vi "Close.vi"(8 "error in (no error)":errorcluster, 11 "DIO Ref In":T1) -> (0 "error out":errorcluster)   [LabVIEW 2021, in "DIO.lvlib"]
doc: "Closes the reference to one or more digital I/O channels, sets the logic levels of all output channels to low, and disables all output channels."
uses:
  <vilib>/myRIO/Instrument Drivers/Onboard IO/DIO/DIO.lvlib
  <vilib>/myRIO/Instrument Drivers/Onboard IO/DIO/typedefs/DIO Reference.ctl
  <vilib>/myRIO/Common/Instrument Driver Framework/Utilities/typedefs/myRIO Generic Hardware Reference.ctl
  <vilib>/myRIO/Common/Instrument Driver Framework/Utilities/typedefs/Hardware Version Enum.ctl
  <vilib>/myRIO/Common/Instrument Driver Framework/Utilities/typedefs/myRIO v1.0 Reference.ctl
  <vilib>/myRIO/Common/Instrument Driver Framework/Utilities/typedefs/Generic FPGA Reference.ctl
  <vilib>/myRIO/Common/Instrument Driver Framework/myRIO v1.0/DIO/typedefs/DIO Channels List.ctl
  <vilib>/myRIO/Common/Instrument Driver Framework/myRIO v1.0/DIO/typedefs/DIO Channels Enum.ctl
  <vilib>/myRIO/Common/Instrument Driver Framework/myRIO v1.0/DIO/vis/myRIO v1.0 Unreserve DIO.vi
  <vilib>/myRIO/Common/Instrument Driver Framework/roboRIO v1.0/DIO/vis/roboRIO v1.0 Unreserve DIO.vi
  <vilib>/myRIO/Common/Instrument Driver Framework/ELVIS III v1.0/DIO/vis/ELVIS III v1.0 Unreserve DIO.vi
  <vilib>/myRIO/Common/Instrument Driver Framework/myRIO v1.0/DIO/vis/myRIO v1.0 Build MUX Configuration DIO.vi
  <vilib>/myRIO/Common/Instrument Driver Framework/myRIO v1.0/Resource Manager/vis/myRIO v1.0 Unreserve Channel List.vi
  <vilib>/myRIO/Common/Instrument Driver Framework/roboRIO v1.0/Resource Manager/vis/roboRIO v1.0 Unreserve Channel List.vi
  <vilib>/myRIO/Common/Instrument Driver Framework/roboRIO v1.0/DIO/vis/roboRIO v1.0 Build MUX Configuration DIO.vi
  <vilib>/myRIO/Common/Instrument Driver Framework/ELVIS III v1.0/DIO/vis/ELVIS III v1.0 Build MUX Configuration DIO.vi
  <vilib>/myRIO/Common/Instrument Driver Framework/myRIO v1.0/Resource Manager/vis/myRIO v1.0 Create Configuration List.vi
  <vilib>/myRIO/Common/Instrument Driver Framework/myRIO v1.0/Resource Manager/vis/myRIO v1.0 Unreserve Channel.vi
  <vilib>/myRIO/Common/Instrument Driver Framework/roboRIO v1.0/Resource Manager/vis/roboRIO v1.0 Unreserve Channel.vi
  <vilib>/myRIO/Common/Instrument Driver Framework/roboRIO v1.0/Resource Manager/vis/roboRIO v1.0 Create Configuration List.vi
  <vilib>/myRIO/Common/Instrument Driver Framework/ELVIS III v1.0/Resource Manager/vis/ELVIS III v1.0 Create Configuration List.vi
  <vilib>/myRIO/Common/Instrument Driver Framework/myRIO v1.0/Resource Manager/vis/myRIO v1.0 Build Mutex Name.vi
  <vilib>/myRIO/Common/Instrument Driver Framework/roboRIO v1.0/Resource Manager/vis/roboRIO v1.0 Build Mutex Name.vi
  <vilib>/myRIO/Common/Instrument Driver Framework/myRIO v1.0/DIO/vis/myRIO v1.0 Shutdown DIO.vi
  <vilib>/myRIO/Common/Instrument Driver Framework/myRIO v1.0/Resource Manager/vis/myRIO v1.0 Configure IO.vi
  <vilib>/myRIO/Common/Instrument Driver Framework/Utilities/vis/Configuration Manager.vi
  <vilib>/myRIO/Common/Instrument Driver Framework/Utilities/vis/IO Manager.vi
  <vilib>/myRIO/Common/Instrument Driver Framework/roboRIO v1.0/DIO/vis/roboRIO v1.0 Shutdown DIO.vi
  <vilib>/myRIO/Common/Instrument Driver Framework/roboRIO v1.0/Resource Manager/vis/roboRIO v1.0 Configure IO.vi
  <vilib>/myRIO/Common/Instrument Driver Framework/ELVIS III v1.0/DIO/vis/ELVIS III v1.0 Shutdown DIO.vi
  <vilib>/myRIO/Common/Instrument Driver Framework/ELVIS III v1.0/Resource Manager/vis/ELVIS III v1.0 Configure IO.vi
  <vilib>/myRIO/Common/Instrument Driver Framework/ELVIS III v1.0/Resource Manager/vis/ELVIS III v1.0 Unreserve Channel List.vi
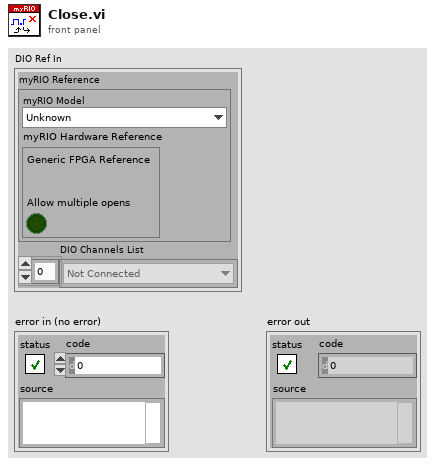
[diagram p1: front panel]
types:
  T1 = typedef "DIO.lvlib/DIO Reference.ctl" = cluster{"myRIO Reference":T2, "DIO Channels List":T6}
  T2 = typedef "myRIO Generic Hardware Reference.ctl" = cluster{"myRIO Model":T3, "myRIO Hardware Reference":T4}
  T3 = typedef "Hardware Version Enum.ctl" = enum16{"Unknown", "myRIO-1900", "myRIO-1950", "roboRIO", "NI ELVIS RIO CM", "ELVIS III"}
  T4 = typedef "myRIO v1.0 Reference.ctl" = cluster{"Generic FPGA Reference":T5, "Allow multiple opens":bool}
  T5 = typedef "Generic FPGA Reference.ctl" = refnum<k20>
  T6 = typedef "DIO Channels List.ctl" = T7[]
  T7 = typedef "DIO Channels Enum.ctl" = enum16{"Not Connected", "C/DIO0", "C/DIO1", "C/DIO2", "C/DIO3", "C/DIO4", "C/DIO5", "C/DIO6", "C/DIO7", "A/DIO0", "A/DIO1", "A/DIO2", "A/DIO3", "A/DIO4", "A/DIO5", "A/DIO6", "A/DIO7", "A/DIO8", "A/DIO9", "A/DIO10", "A/DIO11", "A/DIO12", "A/DIO13", "A/DIO14", "A/DIO15", "A/DIO16", "A/DIO17", "A/DIO18", "A/DIO19", "B/DIO0", "B/DIO1", "B/DIO2", "B/DIO3", "B/DIO4", "B/DIO5", "B/DIO6", "B/DIO7", "B/DIO8", "B/DIO9", "B/DIO10", "B/DIO11", "B/DIO12", "B/DIO13", "B/DIO14", "B/DIO15", "B/DIO16", "B/DIO17", "B/DIO18", "B/DIO19", "LED0", "LED1", "LED2", "LED3", "Button0", "DIO/DIO0", "DIO/DIO1", "DIO/DIO2", "DIO/DIO3", "DIO/DIO4", "DIO/DIO5", "DIO/DIO6", "DIO/DIO7", "DIO/DIO8", "DIO/DIO9", "SPI/CS0", "SPI/CS1", "SPI/CS2", "SPI/CS3", "LED RADIO (Green)", "LED RADIO (Red)", "LED COMM (Green)", "LED COMM (Red)", "LED MODE (Green)", "LED MODE (Red)"}
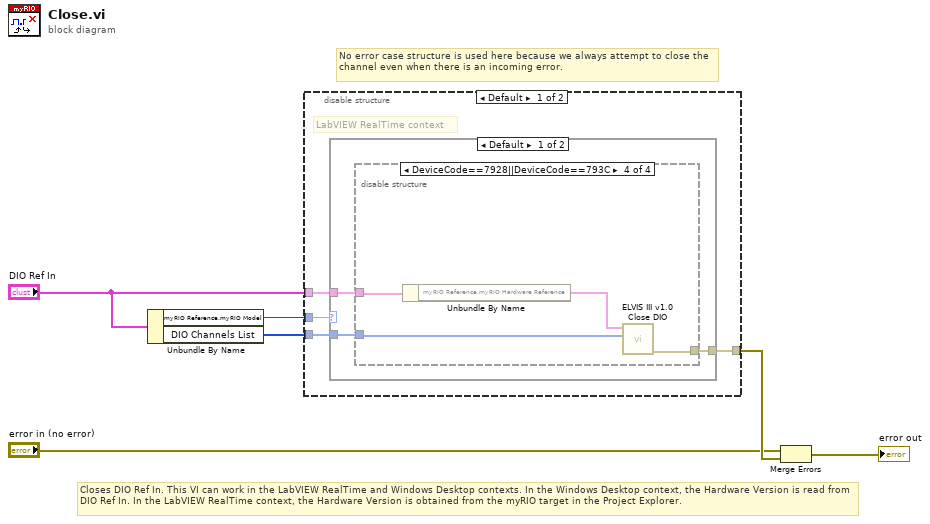
[diagram p0: block diagram]
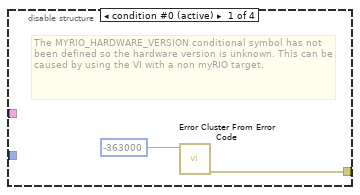
[diagram p2: hidden frame]
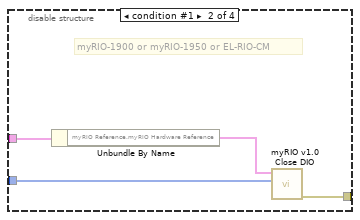
[diagram p3: hidden frame]
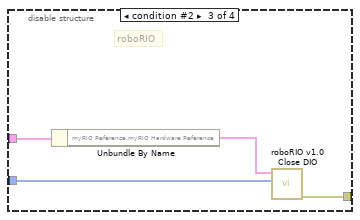
[diagram p4: hidden frame]
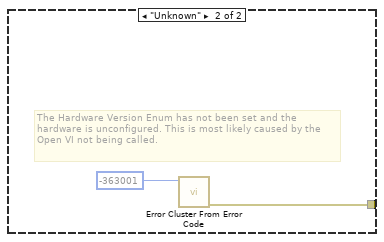
[diagram p5: hidden frame]
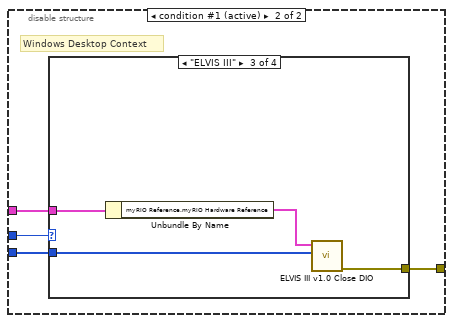
[diagram p6: hidden frame]
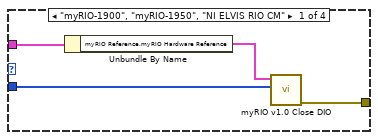
[diagram p7: hidden frame]
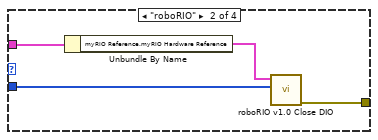
[diagram p8: hidden frame]
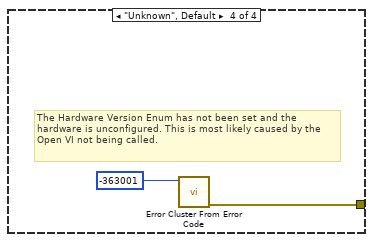
[diagram p9: hidden frame]
diagram:
  # "No error case structure is used here because we always attempt to close the channel even when there is an incoming error."
  # "Closes DIO Ref In. This VI can work in the LabVIEW RealTime and Windows Desktop contexts. In the Windows Desktop context, the Hardware Version is read from DIO Ref In. In the LabVIEW RealTime context, the Hardware Version is obtained from the myRIO target in the Project Explorer."
  n1 = Unbundle By Name("DIO Ref In") -> ("myRIO Reference.myRIO Model"=w2:T3, "DIO Channels List"=w1:T6)
  n2 = disable-structure shown="Default" {
    disable-tunnel: [w10 w33] -> w6
    disable-tunnel: "DIO Ref In" -> [w9 w32]
    disable-tunnel: w2 -> [w8 w31]
    disable-tunnel: w1 -> [w7 w30]
    frame condition #0 {
      # "LabVIEW RealTime context"
      n3 = case shown="Default" w8 {
        tunnel: w9 -> [w13 _]
        tunnel: [w12 w28] -> w10
        tunnel: w7 -> [w11 _]
        frame Default {
          n4 = disable-structure shown="DeviceCode==7928||DeviceCode==793C" {
            disable-tunnel: w13 -> [_ w16 w20 w26]
            disable-tunnel: [w14 w19 w23 w24] -> w12
            disable-tunnel: w11 -> [_ w17 w21 w25]
            frame condition #0 (active) {
              # "The MYRIO_HARDWARE_VERSION conditional symbol has not been defined so the hardware version is unknown. This can be caused by using the VI with a non myRIO target."
              n5 = call <vilib>:"Error Cluster From Error Code.vi"("error code (0)"=-363000) -> ("error out"=w14:errorcluster)  [unwired: 8 in]
            }
            frame condition #1 {
              # "myRIO-1900 or myRIO-1950 or EL-RIO-CM"
              n6 = Unbundle By Name(w16) -> ("myRIO Reference.myRIO Hardware Reference"=w18:T4)
              n7 = call <vilib>:"myRIO v1.0 Close DIO.vi"("DIO Channel List"=w17, "myRIO Ref In"=w18) -> ("error out"=w19:errorcluster)  [unwired: 9 in]
            }
            frame condition #2 {
              # "roboRIO"
              n8 = Unbundle By Name(w20) -> ("myRIO Reference.myRIO Hardware Reference"=w22:T4)
              n9 = call <vilib>:"roboRIO v1.0 Close DIO.vi"("DIO Channel List"=w21, "myRIO Ref In"=w22) -> ("error out"=w23:errorcluster)  [unwired: 9 in]
            }
            frame condition #3 {
              n10 = Unbundle By Name(w26) -> ("myRIO Reference.myRIO Hardware Reference"=w27:T4)
              n11 = call <vilib>:"ELVIS III v1.0 Close DIO.vi"("DIO Channel List"=w25, "myRIO Ref In"=w27) -> ("error out"=w24:errorcluster)  [unwired: 9 in]
            }
          }
        }
        frame "Unknown" {
          # "The Hardware Version Enum has not been set and the hardware is unconfigured. This is most likely caused by the Open VI not being called."
          n12 = call <vilib>:"Error Cluster From Error Code.vi"("error code (0)"=-363001) -> ("error out"=w28:errorcluster)  [unwired: 8 in]
        }
      }
    }
    frame condition #1 (active) {
      # "Windows Desktop Context"
      n13 = case shown="\"ELVIS III\"" w31 {
        tunnel: w32 -> [w34 w38 w44 _]
        tunnel: [w37 w41 w42 w46] -> w33
        tunnel: w30 -> [w36 w40 w43 _]
        frame "myRIO-1900", "myRIO-1950", "NI ELVIS RIO CM" {
          n14 = Unbundle By Name(w34) -> ("myRIO Reference.myRIO Hardware Reference"=w35:T4)
          n15 = call <vilib>:"myRIO v1.0 Close DIO.vi"("DIO Channel List"=w36, "myRIO Ref In"=w35) -> ("error out"=w37:errorcluster)  [unwired: 9 in]
        }
        frame "roboRIO" {
          n16 = Unbundle By Name(w38) -> ("myRIO Reference.myRIO Hardware Reference"=w39:T4)
          n17 = call <vilib>:"roboRIO v1.0 Close DIO.vi"("DIO Channel List"=w40, "myRIO Ref In"=w39) -> ("error out"=w41:errorcluster)  [unwired: 9 in]
        }
        frame "ELVIS III" {
          n18 = Unbundle By Name(w44) -> ("myRIO Reference.myRIO Hardware Reference"=w45:T4)
          n19 = call <vilib>:"ELVIS III v1.0 Close DIO.vi"("DIO Channel List"=w43, "myRIO Ref In"=w45) -> ("error out"=w42:errorcluster)  [unwired: 9 in]
        }
        frame "Unknown", Default {
          # "The Hardware Version Enum has not been set and the hardware is unconfigured. This is most likely caused by the Open VI not being called."
          n20 = call <vilib>:"Error Cluster From Error Code.vi"("error code (0)"=-363001) -> ("error out"=w46:errorcluster)  [unwired: 8 in]
        }
      }
    }
  }
  n21 = Merge Errors("error in (no error)", w6) -> (→"error out":errorcluster)
